vi "RampRateSingle.vi"(6 "return immediately":bool, 8 "error in (no error)":T1, 9 "ramp rate":dbl, 10 "axis name":string, 11 "controller In":refnum<k24>) -> (0 "error Out":T1, 3 "controller out":refnum<k24>)   [LabVIEW 2013]
doc: "Acceleration and Deceleration rates are set to ramp rate for the specified axis."
uses:
  C:/Program Files (x86)/Aerotech/Ensemble/LabVIEW/8.2/Bin/Aerotech.Ensemble.dll
  Bin/Aerotech.Ensemble.dll
  C:/Program Files (x86)/Aerotech/Ensemble/LabVIEW/8.2/Bin/Aerotech.Ensemble.LabVIEW.dll
  Bin/Aerotech.Ensemble.LabVIEW.dll
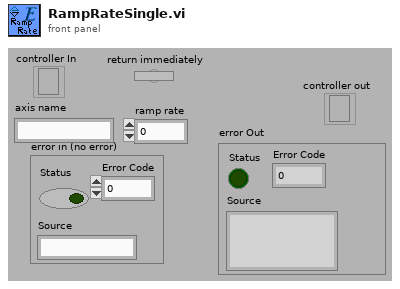
[diagram p1: front panel]
types:
  T1 = cluster{"Status":bool, "Error Code":i32, "Source":string}
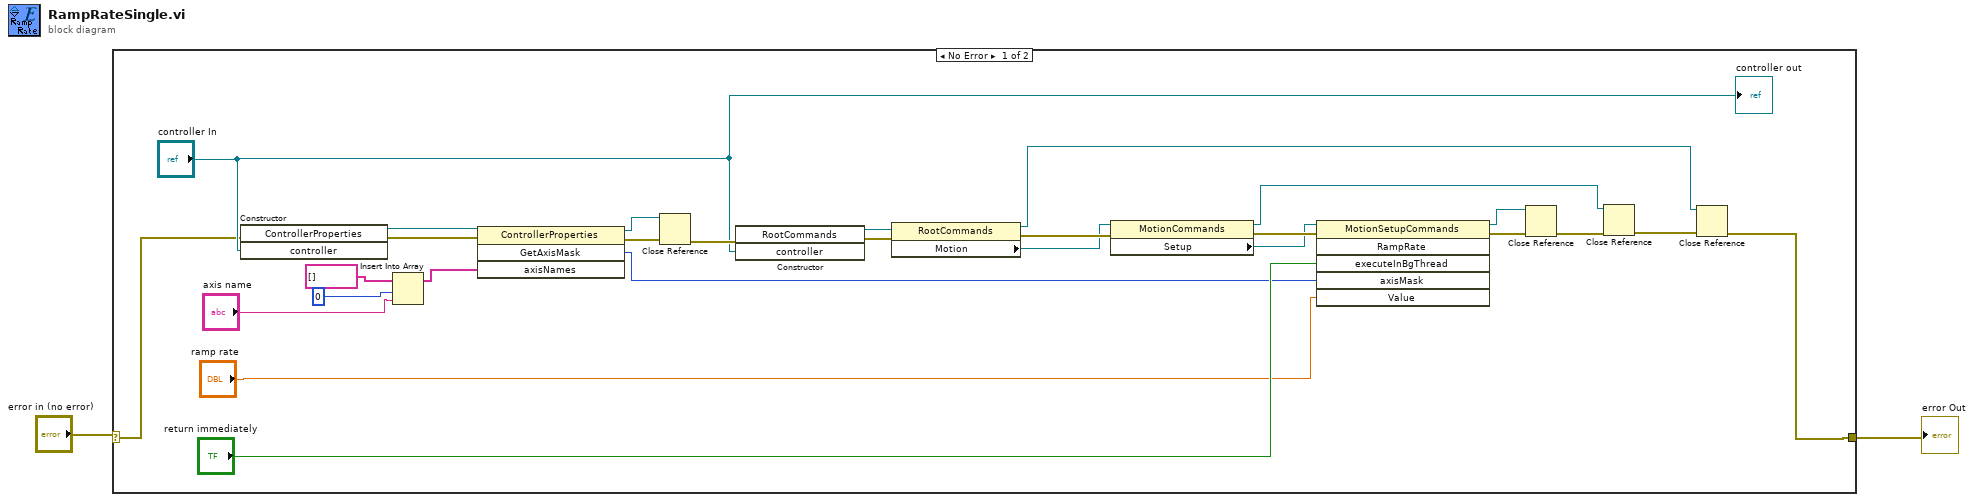
[diagram p0: block diagram]
diagram:
  n1 = case shown="No Error" "error in (no error)" {
    selector: "error in (no error)" -> [w9 w30]
    tunnel: [w8 w30] -> w1
    frame No Error {
      n2 = constructor class="ControllerProperties"(error in=w9, "controller"="controller In") -> (reference out=w28:refnum<k24>, error out=w29:errorcluster)  [unwired: 2 in, 2 out]
      n3 = Insert Into Array(array=string[] [], index=0, new element="axis name") -> (w3:string[])
      n4 = invoke class="ControllerProperties" method="GetAxisMask"(reference=w28, error in=w29, "axisNames"=w3) -> (reference out=w26:refnum<k24>, error out=w27:errorcluster, "GetAxisMask"=w11:i32)  [unwired: 1 in, 1 out]
      n5 = Close Reference(reference=w26, error in (no error)=w27) -> (error out=w25:errorcluster)
      n6 = constructor class="RootCommands"(error in=w25, "controller"="controller In") -> (reference out=w24:refnum<k24>, error out=w23:errorcluster)  [unwired: 2 in, 2 out]
      n7 = property class="RootCommands"(reference=w24, error in=w23) -> (reference out=w13:refnum<k24>, error out=w22:errorcluster, "Motion"=w21:refnum<k24>)
      n8 = property class="MotionCommands"(reference=w21, error in=w22) -> (reference out=w15:refnum<k24>, error out=w20:errorcluster, "Setup"=w19:refnum<k24>)
      n9 = invoke class="MotionSetupCommands" method="RampRate"(reference=w19, error in=w20, "executeInBgThread"="return immediately", "axisMask"=w11, "Value"="ramp rate") -> (reference out=w17:refnum<k24>, error out=w18:errorcluster)  [unwired: 1 in, 4 out]
      n10 = Close Reference(reference=w17, error in (no error)=w18) -> (error out=w16:errorcluster)
      n11 = Close Reference(reference=w15, error in (no error)=w16) -> (error out=w14:errorcluster)
      n12 = Close Reference(reference=w13, error in (no error)=w14) -> (error out=w8:errorcluster)
      "controller out" <- "controller In"
    }
    frame Error {
    }
  }
  "error Out" <- w1
